vi "Write Config File.vi"(11 "Settings":T1) -> (0 "error out":errorcluster, 3 "Settings Out":T1)   [LabVIEW 2018, in "MWWL Verification.lvlib" / "MWWL Verification.lvclass"]
uses:
  MWWL Verification.lvclass
  Type Defs/ConfigSettings.ctl
  <vilib>/Utility/config.llb/Write Key (String).vi
  <vilib>/Utility/config.llb/NI_LVConfig.lvlib
  MWWL Verification.lvlib
panel:
  in  "OK Button":bool
  # "SM140"
  # "SM140"
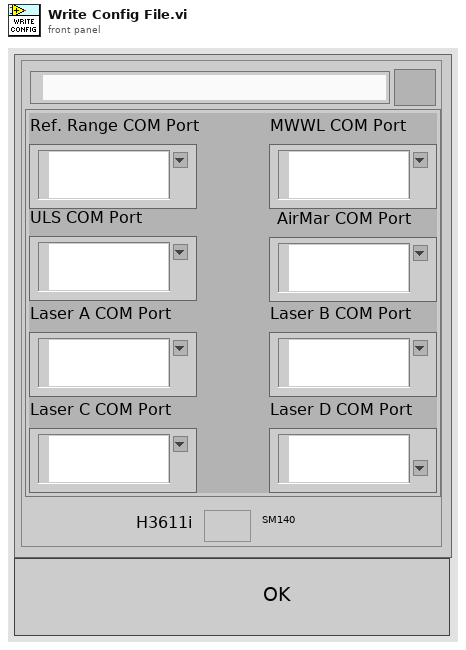
[diagram p1: front panel]
types:
  T1 = typedef "MWWL Verification.lvlib/ConfigSettings.ctl" = cluster{"Base Path":path, "DNL_Configuration Settings.Ports":cluster{"Ref. Range COM Port":refnum<visa-resource-name>, "MWWL COM Port":refnum<visa-resource-name>, "ULS COM Port":refnum<visa-resource-name>, "Laser A COM Port":refnum<visa-resource-name>, "Laser B COM Port":refnum<visa-resource-name>, "Laser C COM Port":refnum<visa-resource-name>, "Laser D COM Port":refnum<visa-resource-name>, "AirMar COM Port":refnum<visa-resource-name>}, "H3611i":bool}
  T2 = cluster{"Ref. Range COM Port":refnum<visa-resource-name>, "MWWL COM Port":refnum<visa-resource-name>, "ULS COM Port":refnum<visa-resource-name>, "Laser A COM Port":refnum<visa-resource-name>, "Laser B COM Port":refnum<visa-resource-name>, "Laser C COM Port":refnum<visa-resource-name>, "Laser D COM Port":refnum<visa-resource-name>, "AirMar COM Port":refnum<visa-resource-name>}
  T3 = typedef "NI_LVConfig.lvlib/Config Data RefNum.ctl" = refnum<k1>
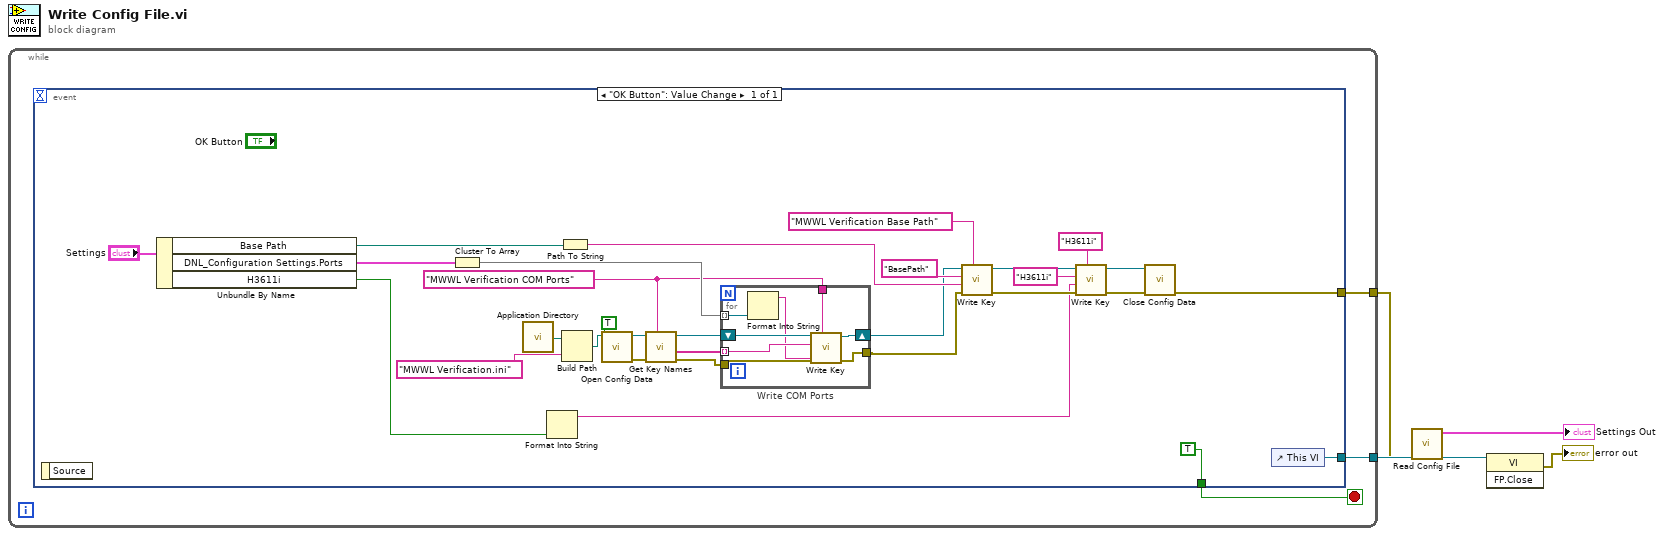
[diagram p0: block diagram]
diagram:
  n1 = while {
    tunnel: [w7] -> w5
    tunnel: [w6] -> w1
    stop <- w8 stop-if-true
    n2 = event shown="[0] \"OK Button\": Value Change" {
      selector: _ -> [_]
      dyn-events: _ -> [_]
      timeout: _ -> [_]
      tunnel: [TRUE] -> w8
      tunnel: [w20] -> w7
      tunnel: [w9] -> w6
      event "OK Button": Value Change {
        w23 = "MWWL Verification COM Ports" ("section")
        n3 = event-data() -> ()  [unwired: 1 in, 1 out]
        n4 = Unbundle By Name("Settings") -> ("Base Path"=w38:path, "DNL_Configuration Settings.Ports"=w37:T2, "H3611i"=w12:bool)
        n5 = Cluster To Array(cluster=w37) -> (array=w32:refnum<visa-resource-name>[])
        n6 = call <vilib>:"Application Directory.vi"() -> ("Application Directory"=w36:path)
        n7 = Format Into String(w12) -> (resulting string=w11:string)  [unwired: 3 in, 1 out]
        n8 = Path To String(path=w38) -> (string=w28:string)
        n9 = Build Path(base path=w36, name or relative path="MWWL Verification.ini") -> (appended path=w34:path)
        n10 = call <vilib>:"Open Config Data.vi"("create file if necessary (T)"=TRUE, "configuration file path"=w34) -> ("error out"=w21:errorcluster, "refnum"=w31:T3)  [unwired: 7 in, 1 out]
        n11 = call <vilib>:"Get Key Names.vi"("section"=w23, "error in (no error)"=w21, "refnum"=w31) -> ("error out"=w22:errorcluster, "key names"=w30:string[], "refnum out"=w29:T3)  [unwired: 5 in, 1 out]
        n12 = for "Write COM Ports" {
          tunnel: w32 -> [w46] mode=indexing
          tunnel: w30 -> [w44] mode=indexing
          tunnel: [w42] -> w24
          shift-right: [w41] -> w25
          shift-left: w29 -> [w45]
          tunnel: w23 -> [w40]
          tunnel: w22 -> [w39]
          n13 = Format Into String(w46) -> (resulting string=w43:string)  [unwired: 3 in, 1 out]
          n14 = call-poly <vilib>:"Write Key.vi"("section"=w40, "error in (no error)"=w39, "value"=w43, "key"=w44, "refnum"=w45) -> ("error out"=w42:errorcluster, "refnum out"=w41:T3)  [unwired: 4 in, 1 out]
        }
        n15 = call-poly <vilib>:"Write Key.vi"("section"="MWWL Verification Base Path", "error in (no error)"=w24, "value"=w28, "key"="BasePath" ("section"), "refnum"=w25) -> ("error out"=w16:errorcluster, "refnum out"=w18:T3)  [unwired: 4 in, 1 out]
        n16 = call-poly <vilib>:"Write Key.vi"("section"="H3611i", "error in (no error)"=w16, "value"=w11, "key"="H3611i" ("section"), "refnum"=w18) -> ("error out"=w15:errorcluster, "refnum out"=w17:T3)  [unwired: 4 in, 1 out]
        n17 = call <vilib>:"Close Config Data.vi"("error in (no error)"=w15, "refnum"=w17) -> ("error out"=w9:errorcluster)  [unwired: 8 in, 1 out]
        n18 = control-ref of="This VI"() -> (w20:refnum<vi>)
      }
    }
  }
  n19 = call "Read Config File.vi"("error in (no error)"=w1) -> ("error out"=w2:errorcluster, "Settings Out"=→"Settings Out":T1)  [unwired: 9 in]
  n20 = invoke class="VI" method="FP.Close"(reference=w5, error in=w2) -> (error out=→"error out":errorcluster)  [unwired: 1 in, 2 out]
